vi "Read Number of Row Items.vi"(8 "error in (no error)":errorcluster, 11 "AdjustableMulticolumnListbox in":refnum<class "AdjMCLB.lvclass">) -> (0 "error out":errorcluster, 2 "Rows":i32, 3 "AdjustableMulticolumnListbox out":refnum<class "AdjMCLB.lvclass">)   [LabVIEW 2020, in "AdjMCLB.lvclass"]
uses:
  AdjMCLB.lvclass
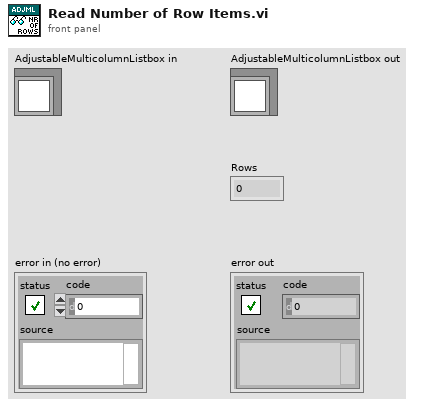
[diagram p1: front panel]
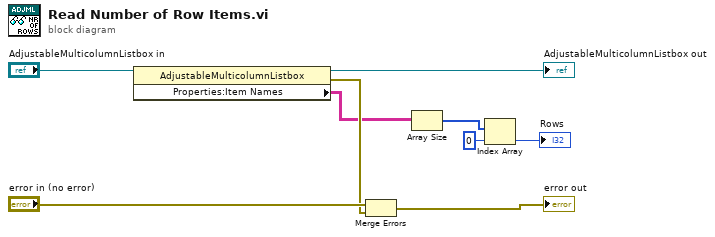
[diagram p0: block diagram]
diagram:
  n1 = property class="AdjustableMulticolumnListbox"(reference="AdjustableMulticolumnListbox in") -> (reference out=→"AdjustableMulticolumnListbox out":refnum<class "AdjMCLB.lvclass">, error out=w5:errorcluster, "Properties:Item Names"=w4:string[][])  [unwired: 1 in]
  n2 = Merge Errors("error in (no error)", w5) -> (→"error out":errorcluster)
  n3 = Array Size(array=w4) -> (size(s)=w3:i32[])
  n4 = Index Array(array=w3, index=0) -> (element=→"Rows":i32)
